vi "Write to File.vi"(8 "error in":errorcluster, 10 "File Actor In":refnum<class "File Actor.lvclass">, 11 "Exe Write Taus in":refnum<class "Exe Write Taus.lvclass">) -> (0 "error out":errorcluster, 2 "File Actor Out":refnum<class "File Actor.lvclass">)   [LabVIEW 2014]
doc: "This is the sould of the execution method and the only VI that should be overriden. This is where we expect the file to be written."
uses:
  reusable/Session APIs/Session Log/System Log.lvclass
  reusable/Data/Data.lvclass
  reusable/PAS/Data/Main/PAS Data.lvclass
  File Actor/File Actor.lvclass
  reusable/PAS/Data/Cell/PAS Cell Data.lvclass
  Exe Write Taus.lvclass
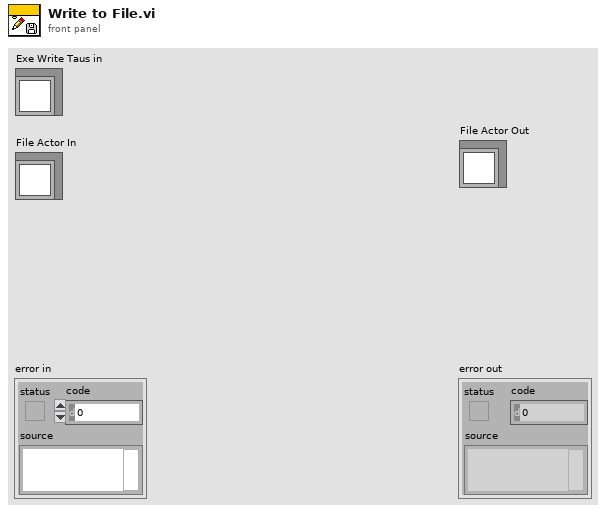
[diagram p1: front panel]
types:
  T1 = typedef "Session - Root.lvclass/Session Handle.ctl" = refnum<data-value>
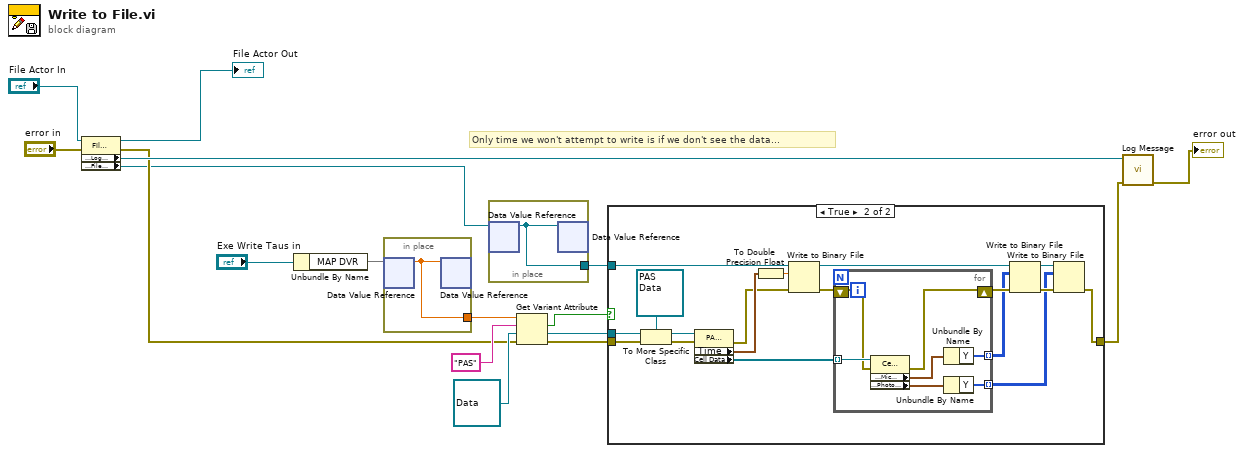
[diagram p0: block diagram]
diagram:
  # "Only time we won't attempt to write is if we don't see the data..."
  n1 = property class="File Actor"(reference="File Actor In", error in="error in") -> (reference out=→"File Actor Out":refnum<class "File Actor.lvclass">, error out=w8:errorcluster, "Accessors:Log Session"=w15:T1, "Accessors:File DVR"=w7:refnum<data-value>)
  n2 = Unbundle By Name("Exe Write Taus in") -> ("MAP DVR"=w1)
  n3 = in-place {
    in-place-border: [w18] -> w16
    n4 = in-place-dvr #1(w1) -> (w18:dbl)  [unwired: 1 out]
    n5 = in-place-dvr #1(w18) -> ()  [unwired: 2 out]
  }
  n6 = in-place {
    in-place-border: [w19] -> w17
    n7 = in-place-dvr #2(w7) -> (w19:refnum<file>)  [unwired: 1 out]
    n8 = in-place-dvr #2(w19) -> ()  [unwired: 2 out]
  }
  n9 = Get Variant Attribute(Variant=w16, name="PAS", default value (empty Variant)=refnum<class "Data.lvclass"> refnum ("Base Data Lib:Data"), error in=w8) -> (found=w10:bool, value=w11:refnum<class "Data.lvclass">, error out=w9:errorcluster)  [unwired: 1 out]
  n10 = case shown="True" w10 {
    tunnel: [w20 w21] -> w14
    tunnel: w17 -> [_ w32]
    tunnel: w11 -> [_ w38]
    tunnel: w9 -> [w20 w30]
    frame False {
    }
    frame True {
      n11 = To More Specific Class(target class=refnum<class "PAS Data.lvclass"> refnum ("PAS Library.lvlib:PAS Data"), reference=w38, error in=w30) -> (specific class reference=w36:refnum<class "PAS Data.lvclass">, error out=w29:errorcluster)
      n12 = property class="PAS Data"(reference=w36, error in=w29) -> (error out=w28:errorcluster, "Time"=w34:timestamp, "Cell Data"=w35:refnum<class "PAS Cell Data.lvclass">[])  [unwired: 1 out]
      n13 = To Double Precision Float(number=w34) -> (double precision float=w33:dbl)
      n14 = Write to Binary File(file (use dialog)=w32, data=w33, error in=w28) -> (refnum out=w26:refnum<file>, error out=w31:errorcluster)  [unwired: 3 in, 1 out]
      n15 = for {
        tunnel: w35 -> [w45] mode=indexing
        shift-right: [w41] -> w27
        shift-left: w31 -> [w44]
        tunnel: [w40] -> w25 mode=indexing
        tunnel: [w39] -> w22 mode=indexing
        n16 = property class="Cell Data"(reference=w45, error in=w44) -> (error out=w41:errorcluster, "Accessors:Mic Time"=w43:waveform(i16), "Accessors:Photodiode"=w42:waveform(i16))  [unwired: 1 out]
        n17 = Unbundle By Name(w43) -> ("Y"=w40:i16[])
        n18 = Unbundle By Name(w42) -> ("Y"=w39:i16[])
      }
      n19 = Write to Binary File(file (use dialog)=w26, data=w25, error in=w27) -> (refnum out=w24:refnum<file>, error out=w23:errorcluster)  [unwired: 3 in, 1 out]
      n20 = Write to Binary File(file (use dialog)=w24, data=w22, error in=w23) -> (error out=w21:errorcluster)  [unwired: 3 in, 2 out]
    }
  }
  n21 = call "Log Message.vi"("error in"=w14, "session in"=w15) -> ("error out"=→"error out":errorcluster)  [unwired: 8 in, 1 out]
